vi "Write ASCII or Unicode.vi"(8 "error in (no error)":errorcluster, 10 "ASCII or Unicode":T1={"Type"=enum."ASCII", "Direction"=enum."Default"}, 11 "Font Class in":refnum<class "Font Class.lvclass">) -> (0 "error out":errorcluster, 3 "Font Class out":refnum<class "Font Class.lvclass">)   [LabVIEW 2019, in "Font Class.lvclass"]
uses:
  <userlib>/Exaprom PDF/LV Class/Fonts Class/Font Class.lvclass
  <userlib>/Exaprom PDF/Controls/Text Controls/Unicode/Character type with Select.ctl
  <userlib>/Exaprom PDF/Controls/Text Controls/Unicode/Writing direction with Select.ctl
  <userlib>/Exaprom PDF/Controls/Text Controls/Unicode/ASCII or Unicode with Select.ctl
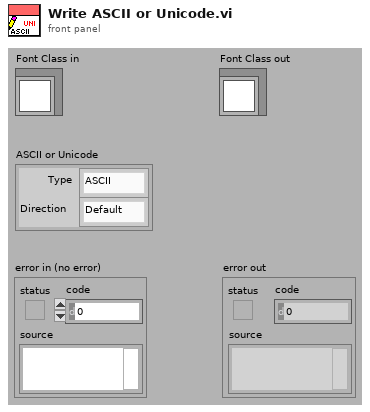
[diagram p1: front panel]
types:
  T1 = typedef "ASCII or Unicode with Select.ctl" = cluster{"Type":T2, "Direction":T3}
  T2 = typedef "Character type with Select.ctl" = enum16{"Select", "ASCII", "Unicode"}
  T3 = typedef "Writing direction with Select.ctl" = enum16{"Select", "Default", "NO BIDI", "LTR", "RTL"}
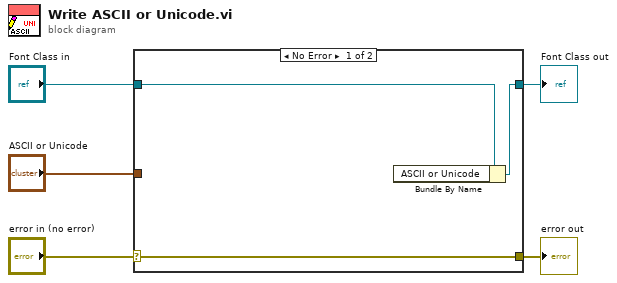
[diagram p0: block diagram]
diagram:
  n1 = case shown="No Error" "error in (no error)" {
    selector: "error in (no error)" -> [w9 w10]
    tunnel: [w9 w10] -> w4
    tunnel: [w7 w11] -> w2
    tunnel: "Font Class in" -> [w8 w11]
    tunnel: "ASCII or Unicode" -> [w6 _]
    frame No Error {
      n2 = Bundle By Name(cluster=w8) -> (w7:refnum<class "Font Class.lvclass">)  [unwired: 1 in]
    }
    frame Error {
    }
  }
  "error out" <- w4
  "Font Class out" <- w2
